vi "Servo MSMT Configure External Network.vi"(8 "error in (no error)":errorcluster, 11 "Servo MSMT in":refnum<class "Servo MSMT.lvclass">) -> (0 "error out":errorcluster, 3 "Servo MSMT out":refnum<class "Servo MSMT.lvclass">)   [LabVIEW 2016]
uses:
  Plugins/QPA Measurement.lvlibp/QPA Measurement.lvclass
  Servo MSMT.lvclass
  Plugins/QPA Measurement.lvlibp/Controls/LoadPull State.ctl
  Plugins/QPA Measurement.lvlibp/Controls/External Network Parameters.ctl
  Plugins/String Database.lvlibp/String Database.lvclass
  C:/Sequence Automation/Plugins/Measurement Interface.lvlibp/Measurement Interface.lvclass
  C:/Sequence Automation/Plugins/FPF.lvlibp/Factory Plugin Framework.lvclass
  Plugins/Measurement Interface.lvlibp/Measurement Interface.lvclass
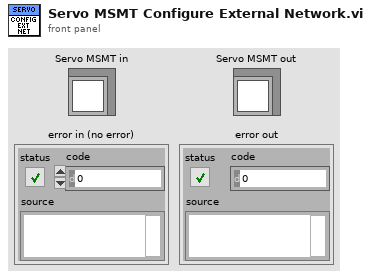
[diagram p1: front panel]
types:
  T1 = typedef "QPA Measurement.lvlibp/QPA Measurement.lvclass/LoadPull State.ctl" = enum16{"Disabled", "Coupled Path", "Uncoupled Path", "Auto"}
  T2 = typedef "QPA Measurement.lvlibp/QPA Measurement.lvclass/External Network Parameters.ctl" = cluster{"LoadPull State":T1, "SG Pin":string, "SA Pin":string, "SG Frequency":dbl, "SA Fundamental Frequency":dbl, "SG Path Name":string, "SG Sub Path Name":string, "SA Path Name":string, "SA Sub Path Name":string, "SA Measure Frequency":dbl}
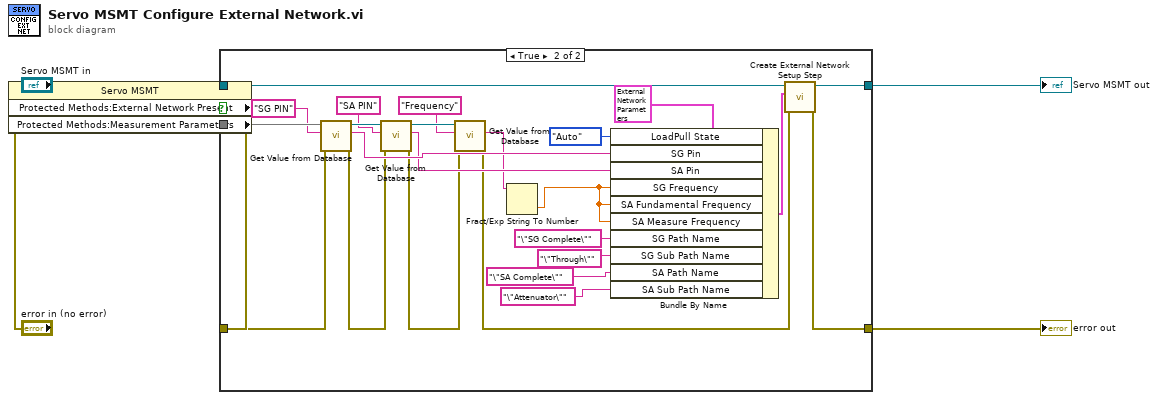
[diagram p0: block diagram]
diagram:
  n1 = property class="Servo MSMT"(reference="Servo MSMT in", error in="error in (no error)") -> (reference out=w3:refnum<class "Servo MSMT.lvclass">, error out=w5:errorcluster, "Protected Methods:External Network Present"=w2, "Protected Methods:Measurement Parameters"=w1)
  n2 = case shown="True" w2 {
    tunnel: [w10 w34] -> w8
    tunnel: [w9 w33] -> w7
    tunnel: w5 -> [w9 w27]
    tunnel: w3 -> [w10 w32]
    tunnel: w1 -> [_ w28]
    frame False {
    }
    frame True {
      n3 = call "Get Value from Database.vi"("error in (no error)"=w27, "Entry Name"="SG PIN", "Message in"=w28) -> ("error out"=w23:errorcluster, "Entry Value"=w25:string, "Message out"=w24:refnum<class "String Database.lvclass">)  [unwired: 5 in, 1 out]
      n4 = call "Get Value from Database.vi"("error in (no error)"=w23, "Entry Name"="SA PIN", "Message in"=w24) -> ("error out"=w19:errorcluster, "Entry Value"=w21:string, "Message out"=w20:refnum<class "String Database.lvclass">)  [unwired: 5 in, 1 out]
      n5 = call "Get Value from Database.vi"("error in (no error)"=w19, "Entry Name"="Frequency", "Message in"=w20) -> ("error out"=w18:errorcluster, "Entry Value"=w16:string)  [unwired: 5 in, 2 out]
      n6 = Fract/Exp String To Number(string=w16) -> (number=w15:dbl)  [unwired: 3 in, 1 out]
      n7 = Bundle By Name(cluster=T2 {"LoadPull State"=enum."Disabled", "SG Pin"="", "SA Pin"="", "SG Frequency"=0.0, "SA Fundamental Frequency"=0.0, "SG Path Name"="", "SG Sub Path Name"="", "SA Path Name"="", "SA Sub Path Name"="", "SA Measure Frequency"=0.0} ("External Network Parameters"), "LoadPull State"=LoadPull_State."Auto", "SG Pin"=w25, "SA Pin"=w21, "SG Frequency"=w15, "SA Fundamental Frequency"=w15, "SA Measure Frequency"=w15, "SG Path Name"="\"SG Complete\"", "SG Sub Path Name"="\"Through\"" ("SG Path Name"), "SA Path Name"="\"SA Complete\"" ("SG Path Name"), "SA Sub Path Name"="\"Attenuator\"" ("SG Path Name")) -> (w30:T2)
      n8 = call "Create External Network Setup Step.vi"("error in (no error)"=w18, "External Network Parameters"=w30, "QPA Measurement in"=w32) -> ("error out"=w33:errorcluster, "QPA Measurement out"=w34:refnum<class "QPA Measurement.lvclass">)  [unwired: 7 in]
    }
  }
  "Servo MSMT out" <- w8
  "error out" <- w7
